vi "Get SMO Database Paths.vi"(5 "getAll Cluster":variant, 7 "Default Paths":string, 8 "error in (no error)":errorcluster, 11 "instrument.PPMS2 in":refnum<class "instrument.PPMS2.lvclass">) -> (0 "error out":errorcluster, 2 "Paths":string, 3 "instrument.PPMS2 out":refnum<class "instrument.PPMS2.lvclass">)   [LabVIEW 2019, in "instrument.PPMS2.lvclass"]
uses:
  instrument.PPMS2.lvclass
  instrument.PPMS/instrument.PPMS.lvclass
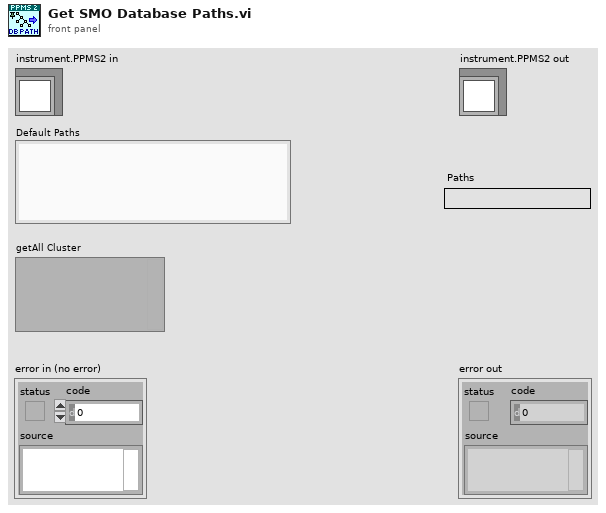
[diagram p1: front panel]
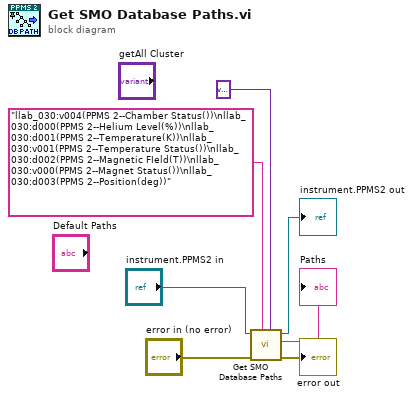
[diagram p0: block diagram]
diagram:
  n1 = call-parent "Get SMO Database Paths.vi"("getAll Cluster"=variant, "Default Paths"="llab_030:v004(PPMS 2--Chamber Status())\nllab_030:d000(PPMS 2--Helium Level(%))\nllab_030:d001(PPMS 2--Temperature(K))\nllab_030:v001(PPMS 2--Temperature Status())\nllab_030:d002(PPMS 2--Magnetic FIeld(T))\nllab_030:v000(PPMS 2--Magnet Status())\nllab_030:d003(PPMS 2--Position(deg))" ("Paths"), "error in (no error)"="error in (no error)", "instrument.PPMS in"="instrument.PPMS2 in") -> ("error out"=→"error out":errorcluster, "Paths"=→"Paths":string, "instrument.PPMS out"=→"instrument.PPMS2 out":refnum<class "instrument.PPMS2.lvclass">)  [unwired: 5 in]
